vi "Create.vi"(7 "gRPC server id":T1, 8 "error in (no error)":errorcluster, 9 "IMeasurementService in":refnum<class "IMeasurementService.lvclass">, 10 "MeasurementPluginService in":refnum<class "MeasurementPluginService.lvclass">, 11 "pin map context":T2) -> (0 "error out":errorcluster, 3 "MeasurementContext out":refnum<class "MeasurementContext.lvclass">)   [LabVIEW 2020, in "MeasurementLink Measurement Server.lvlib" / "MeasurementContext.lvclass"]
uses:
  MeasurementContext.lvclass
  Helpers/TypeDefs/PinMapContext.ctl
  <vilib>/gRPC/LabVIEW gRPC Library/Shared/grpcId.ctl
  IMeasurementService/IMeasurementService.lvclass
  MeasurementPluginService/MeasurementPluginService.lvclass
  Data.ctl
  MeasurementContext.lvclass/MeasurementContext.ctl
  MeasurementLink Measurement Server.lvlib
  <vilib>/gRPC/LabVIEW gRPC Library/grpc-lvsupport-release.lvlib
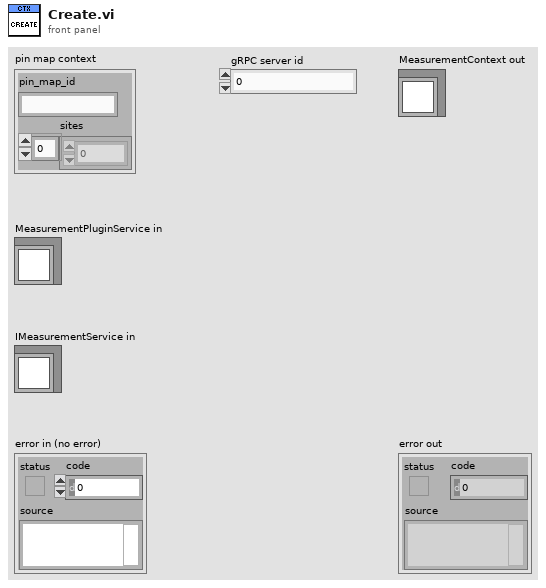
[diagram p1: front panel]
types:
  T1 = typedef "grpc-lvsupport-release.lvlib/grpcId.ctl" = u64
  T2 = typedef "MeasurementLink Measurement Server.lvlib/PinMapContext.ctl" = cluster{"pin_map_id":string, "sites":i32[]}
  T3 = typedef "MeasurementLink Measurement Server.lvlib/MeasurementContext.lvclass/Data.ctl" = cluster{"PinMapContext":T2, "gRPCServerId":T1, "IMeasurementService":refnum<class "IMeasurementService.lvclass">, "MeasurementPluginService":refnum<class "MeasurementPluginService.lvclass">}
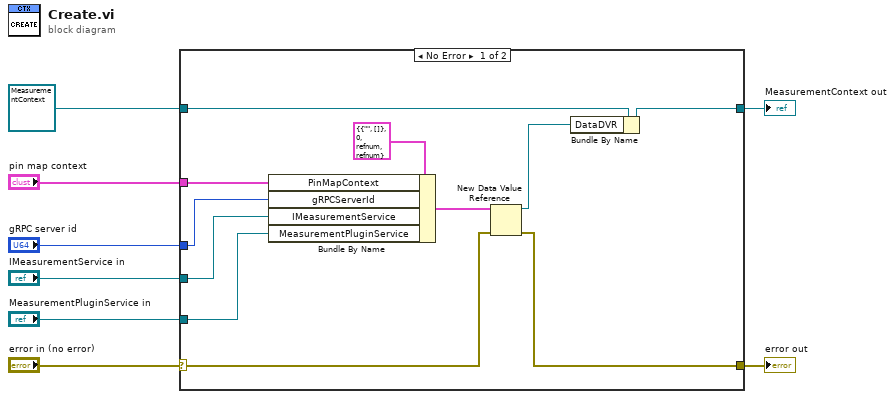
[diagram p0: block diagram]
diagram:
  n1 = case shown="No Error" "error in (no error)" {
    selector: "error in (no error)" -> [w12 w21]
    tunnel: [w9 w21] -> w7
    tunnel: [w18 w20] -> w6
    tunnel: refnum<class "MeasurementContext.lvclass"> refnum ("MeasurementContext.lvclass") -> [w19 w20]
    tunnel: "pin map context" -> [w16 _]
    tunnel: "gRPC server id" -> [w15 _]
    tunnel: "IMeasurementService in" -> [w14 _]
    tunnel: "MeasurementPluginService in" -> [w13 _]
    frame No Error {
      n2 = Bundle By Name(cluster=T3 {"PinMapContext"={"pin_map_id"="", "sites"=[]}, "gRPCServerId"=0, "IMeasurementService"=refnum, "MeasurementPluginService"=refnum} ("Data"), "PinMapContext"=w16, "gRPCServerId"=w15, "IMeasurementService"=w14, "MeasurementPluginService"=w13) -> (w11:T3)
      n3 = New Data Value Reference(data value=w11, error in=w12) -> (data value reference=w10:refnum<data-value>, error out=w9:errorcluster)
      n4 = Bundle By Name(cluster=w19, "DataDVR"=w10) -> (w18:refnum<class "MeasurementContext.lvclass">)
    }
    frame Error {
    }
  }
  "error out" <- w7
  "MeasurementContext out" <- w6
